vi "Serial.vi"(8 "error in (no error)":errorcluster, 9 "Clear Log":bool, 10 "write buffer":string="UA[3]\r\n", 11 "VISA resource name":refnum<visa-resource-name>="COM6") -> (0 "error out":errorcluster, 2 "read buffer":string)   [LabVIEW 2017]
uses:
  <vilib>/Instr/_visa.llb/VISA Configure Serial Port (Instr).vi
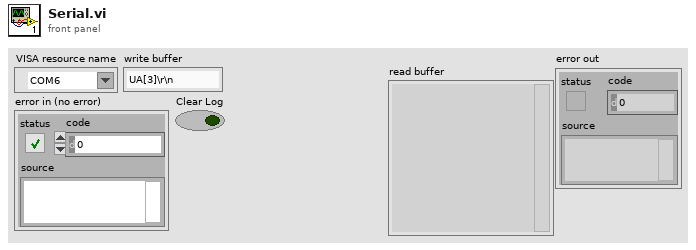
[diagram p1: front panel]
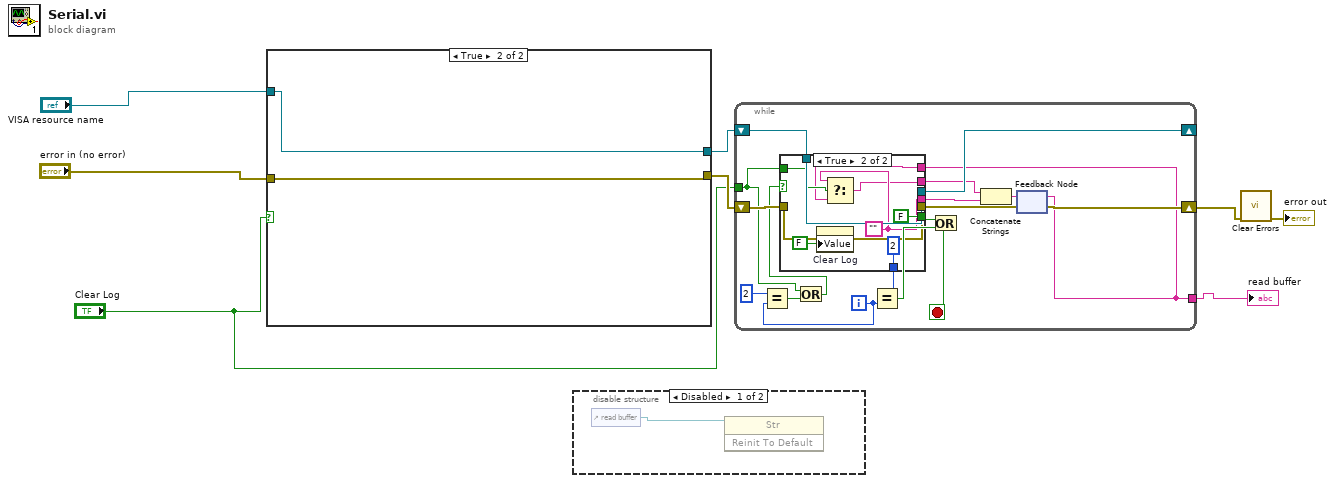
[diagram p0: block diagram]
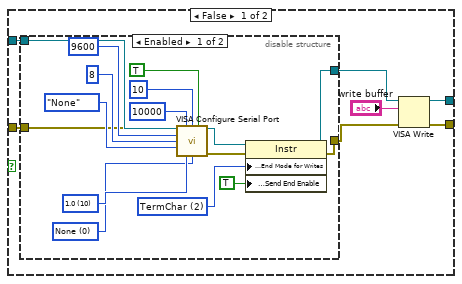
[diagram p3: hidden frame]
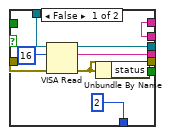
[diagram p5: hidden frame]
diagram:
  n1 = case shown="True" "Clear Log" {
    tunnel: "VISA resource name" -> [w15 w35]
    tunnel: "error in (no error)" -> [w14 w34]
    tunnel: [w11 w35] -> w3
    tunnel: [w10 w34] -> w2
    frame False {
      n2 = disable-structure shown="Enabled" {
        disable-tunnel: w15 -> [w31 w33]
        disable-tunnel: w14 -> [w25 w32]
        disable-tunnel: [w20 w33] -> w12
        disable-tunnel: [w19 w32] -> w13
        frame Enabled {
          w17 = u16 2 items=["None", "LastBit", "TermChar", "Break"] ("Serial Settings:Serial End Mode for Writes")
          w23 = u16 0 items=["None", "XON/XOFF", "RTS/CTS", "XON/XOFF & RTS/CTS", "DTR/DSR", "XON/XOFF & DTR/DSR"] ("flow control (0:none)")
          w24 = u16 10 items=["1.0"=10, "1.5"=15, "2.0"=20] ("stop bits (10: 1 bit)")
          n3 = call-poly "VISA Configure Serial Port"("VISA resource name"=w31, "timeout (10sec)"=u32 10000, "termination char\n(0xA = '\\n' = LF)"=u8 10 ("termination char\n(0xA = '\\n' = LF)"), "Enable Termination\nChar (T)"=TRUE ("Enable Termination\nChar (T)"), "baud rate (9600)"=u32 9600, "data bits (8)"=u16 8, "parity (0:none)"=enum16{"None", "Odd", "Even", "Mark", "Space"}."None", "error in (no error)"=w25, "stop bits (10: 1 bit)"=w24, "flow control (0:none)"=w23) -> ("VISA resource name out"=w21:refnum<visa-resource-name>, "error out"=w22:errorcluster)  [unwired: 4 in]
          n4 = property class="Instr"(reference=w21, error in=w22, "Serial Settings:End Mode for Writes"=w17, "Message Based Settings:Send End Enable"=TRUE) -> (reference out=w20:refnum<visa-resource-name>, error out=w19:errorcluster)
        }
        frame Disabled {
        }
      }
      n5 = VISA Write(VISA resource name=w12, write buffer="write buffer", error in (no error)=w13) -> (VISA resource name out=w11:refnum<visa-resource-name>, error out=w10:errorcluster)  [unwired: 1 out]
    }
    frame True {
    }
  }
  n6 = disable-structure shown="Disabled" {
    frame Disabled {
      n7 = control-ref of="read buffer"() -> (w36:refnum<vi>)
      n8 = invoke class="Str" method="Reinit To Default"(reference=w36) -> ()  [unwired: 2 in, 3 out]
    }
    frame Enabled {
    }
  }
  n9 = while {
    shift-right: [w53] -> _
    shift-left: w3 -> [w47]
    shift-right: [w51] -> w7
    shift-left: w2 -> [w46]
    tunnel: [w44] -> w6
    tunnel: "Clear Log" -> [w37]
    i -> [w41]
    stop <- w49 stop-if-true
    n10 = Equal?(x=2, y=w41) -> (x = y?=w39:bool)
    n11 = Or(x=w37, y=w39) -> (x .or. y?=w38:bool)
    n12 = feedback #1() -> (w44:string)  [unwired: 1 in]
    n13 = case shown="True" w38 {
      tunnel: [w62 w71] -> w53
      tunnel: [w61 w65] -> w52
      tunnel: [w59 w70] -> w51
      tunnel: [w58 FALSE ("status")] -> w48
      tunnel: w47 -> [w57 w71]
      tunnel: w46 -> [w56 w70]
      tunnel: w44 -> [w55 w64]
      tunnel: [w55 w63] -> w43
      tunnel: [2 ("x") 2 ("x")] -> w42
      tunnel: w37 -> [_ w66]
      frame False {
        n14 = VISA Read(VISA resource name=w57, byte count=u32 16, error in (no error)=w56) -> (VISA resource name out=w62:refnum<visa-resource-name>, read buffer=w61:string, error out=w59:errorcluster)  [unwired: 1 out]
        n15 = Unbundle By Name(w59) -> ("status"=w58:bool)
      }
      frame True {
        w65 = ""
        n16 = property on="Clear Log" class="Bool (strict)"("Value"=FALSE ("Clear Log")) -> ()  [unwired: 2 in, 2 out]
        n17 = Select(t=w65, s=w66, f=w64) -> (s? t:f=w63:string)
      }
    }
    n18 = Equal?(x=w42, y=w41) -> (x = y?=w50:bool)
    n19 = Or(x=w48, y=w50) -> (x .or. y?=w49:bool)
    n20 = Concatenate Strings(w43, w52) -> (w45:string)
    n21 = feedback-in #1(w45) -> ()
  }
  "read buffer" <- w6
  n22 = call <vilib>:"Clear Errors.vi"("error in (no error)"=w7) -> ("error out"=→"error out":errorcluster)  [unwired: 5 in, 1 out]
